vi "Change in Bundle Definition.vi"(8 "error in (no error)":errorcluster, 10 "Bundle Definition":T1, 11 "Bundle Builder in":refnum<class "Bundle Builder.lvclass">) -> (0 "error out":errorcluster, 1 "Custom Actions File Names":string[](array[string]), 2 "Product List File Names":string[](array[string]), 3 "Bundle Builder out":refnum<class "Bundle Builder.lvclass">, 4 "Bundle Filename":string)   [LabVIEW 2020, in "Bundle Builder.lvclass"]
uses:
  Bundle Builder.lvclass
  Bundle Builder.lvclass/Bundle Builder.ctl
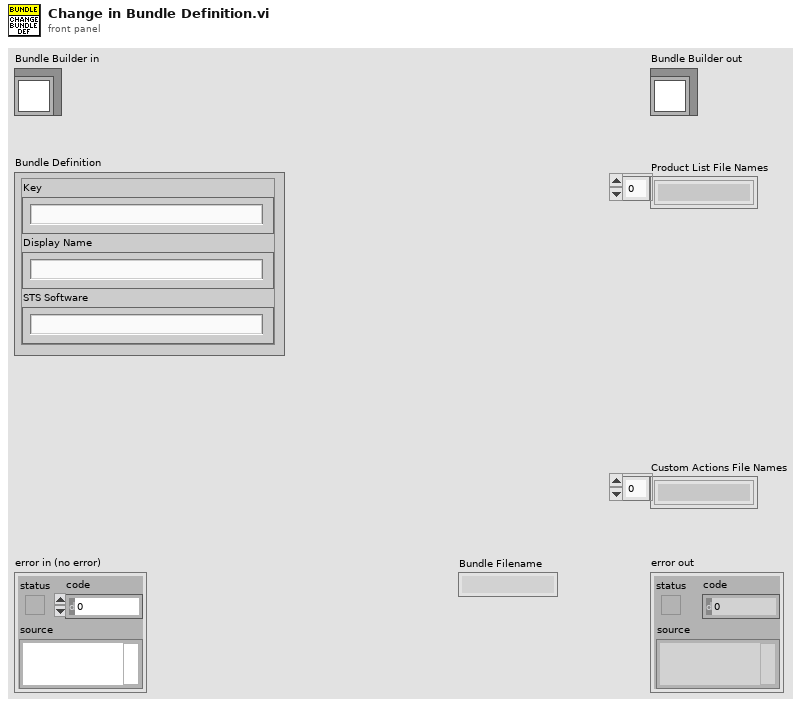
[diagram p1: front panel]
types:
  T1 = cluster{"Key":string, "Display Name":string, "STS Software":string}
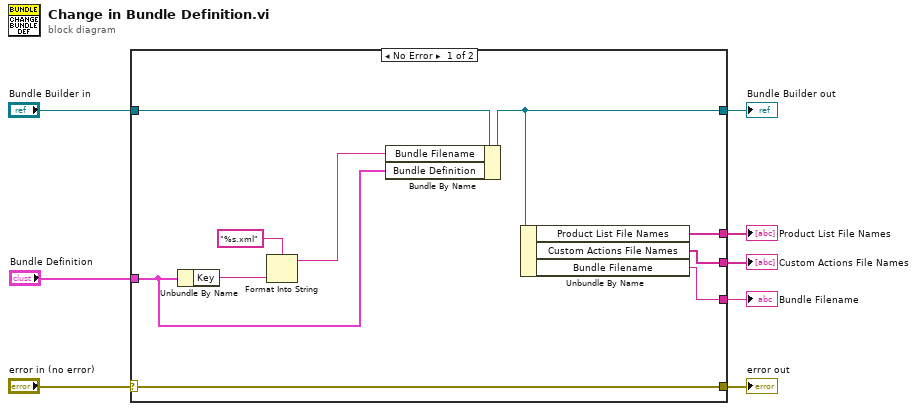
[diagram p0: block diagram]
diagram:
  n1 = case shown="No Error" "error in (no error)" {
    selector: "error in (no error)" -> [w18 w20]
    tunnel: [w18 w20] -> w7
    tunnel: [w16 w19] -> w5
    tunnel: "Bundle Builder in" -> [w17 w19]
    tunnel: "Bundle Definition" -> [w9 _]
    tunnel: [w15 _] -> w4
    tunnel: [w14 _] -> w3
    tunnel: [w13 _] -> w2
    frame No Error {
      n2 = Unbundle By Name(w9) -> ("Key"=w11:string)
      n3 = Format Into String(format string="%s.xml", w11) -> (resulting string=w10:string)  [unwired: 2 in, 1 out]
      n4 = Bundle By Name(cluster=w17, "Bundle Filename"=w10, "Bundle Definition"=w9) -> (w16:refnum<class "Bundle Builder.lvclass">)
      n5 = Unbundle By Name(w16) -> ("Product List File Names"=w15:string[], "Custom Actions File Names"=w14:string[], "Bundle Filename"=w13:string)
    }
    frame Error {
    }
  }
  "error out" <- w7
  "Bundle Builder out" <- w5
  "Product List File Names" <- w4
  "Custom Actions File Names" <- w3
  "Bundle Filename" <- w2
